vi "Host_Simulated Temperature Control.vi"() -> ()   [LabVIEW 2012]
panel:
  out "Stabilized":bool
  in  "stop":bool
  out "Temperature":dbl(slide) scale=0.0..100.0
  in  "Setpoint":dbl=20.0 format="%.2f"
  in  "*Stop_Host*":bool
  in  "Name of RT target":string="localhost"
  in  "TCP Port":u16=12344 min=1025 step=1
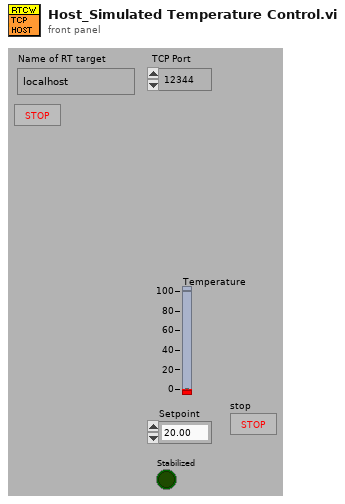
[diagram p1: front panel]
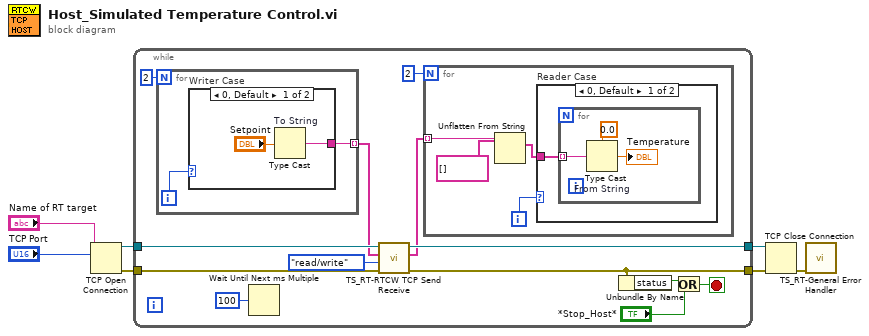
[diagram p0: block diagram]
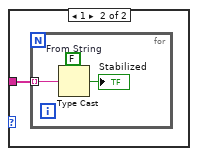
[diagram p2: hidden frame]
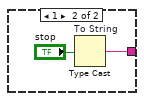
[diagram p3: hidden frame]
diagram:
  n1 = TCP Open Connection(address="Name of RT target", remote port or service name="TCP Port") -> (connection ID=w6:refnum<k5>, error out=w4:errorcluster)  [unwired: 1 in, 2 out]
  n2 = while {
    tunnel: [w19] -> w5
    tunnel: w6 -> [w18]
    tunnel: w4 -> [w20]
    tunnel: [w14] -> w3
    stop <- w12 stop-if-true
    n3 = for {
      N: 2 -> [_]
      tunnel: [w33] -> w16 mode=indexing
      i -> [w34]
      n4 = case "Writer Case" shown="0, Default" w34 {
        tunnel: [w36 w38] -> w33
        frame 0, Default {
          n5 = Type Cast "To String"(x="Setpoint") -> (*(type *) &x=w36:string)  [unwired: 1 out]
        }
        frame 1 {
          n6 = Type Cast "To String"(x="stop") -> (*(type *) &x=w38:string)  [unwired: 1 out]
        }
      }
    }
    n7 = Wait Until Next ms Multiple(millisecond multiple=u32 100) -> ()  [unwired: 1 out]
    n8 = call "TS_RT-RTCW TCP Send Receive.vi"("error in (no error)"=w20, "access (read/write)"=enum16{"read/write", "read only", "write only"}."read/write", "Data In"=w16, "connection ID"=w18) -> ("error out"=w14:errorcluster, "Data Out"=w17:string[], "connection ID Out"=w19:refnum<k5>)  [unwired: 1 out]
    n9 = for {
      N: 2 -> [_]
      tunnel: w17 -> [w22] mode=indexing
      i -> [w24]
      n10 = Unflatten From String(type=string[] [] ("Data Out"), binary string=w22) -> (value=w21:string[])  [unwired: 1 in, 4 out]
      n11 = case "Reader Case" shown="0, Default" w24 {
        tunnel: w21 -> [w25 w29]
        frame 0, Default {
          n12 = for {
            tunnel: w25 -> [w28] mode=indexing
            n13 = Type Cast "From String"(type=0.0 ("Temperature"), x=w28) -> (*(type *) &x=→"Temperature":dbl)
          }
        }
        frame 1 {
          n14 = for {
            tunnel: w29 -> [w32] mode=indexing
            n15 = Type Cast "From String"(type=FALSE ("Stabilized"), x=w32) -> (*(type *) &x=→"Stabilized":bool)
          }
        }
      }
    }
    n16 = Unbundle By Name(w14) -> ("status"=w13:bool)
    n17 = Or(x=w13, y="*Stop_Host*") -> (x .or. y?=w12:bool)
  }
  n18 = TCP Close Connection(connection ID=w5, error in (no error)=w3) -> (error out=w7:errorcluster)  [unwired: 2 out]
  n19 = call "TS_RT-General Error Handler.vi"("error in (no error)"=w7) -> ()  [unwired: 1 in, 14 out]
